vi "zad4.vi"() -> ()   [LabVIEW 2017]
panel:
  in  "Tryb awaryjny":bool
  in  "stop":bool
  out "Lampa Uliczna":cluster{"1":bool, "2":bool, "3":bool}
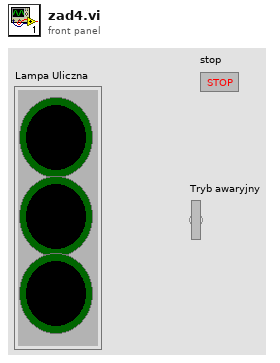
[diagram p1: front panel]
types:
  T1 = cluster{"1":bool, "2":bool, "3":bool, "2":bool, "2":bool, "2":bool, "2":bool, "2":bool}
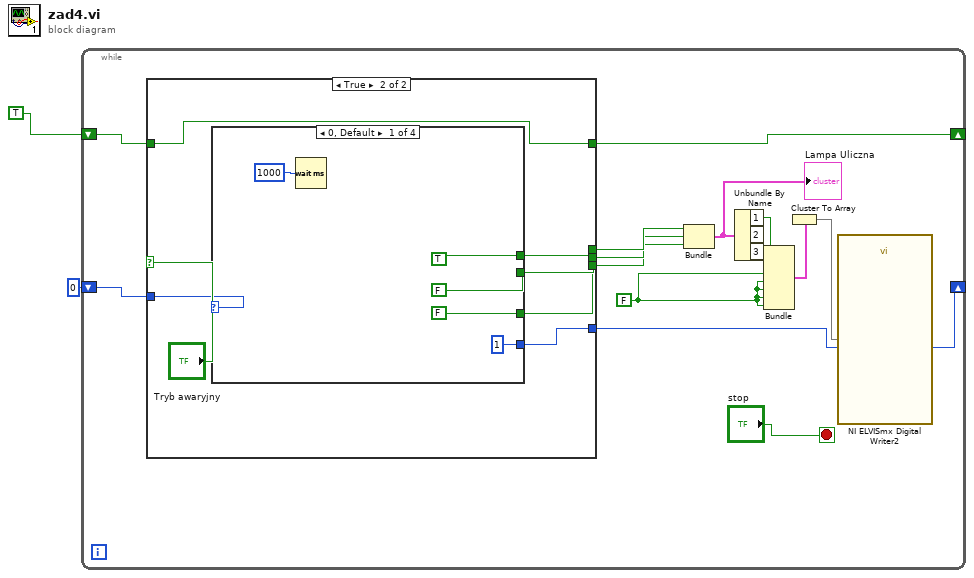
[diagram p0: block diagram]
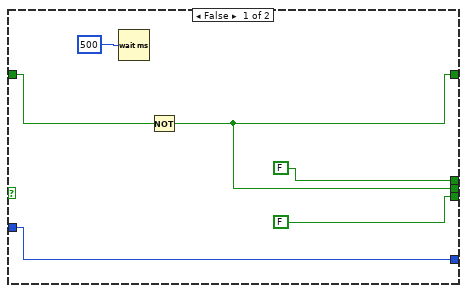
[diagram p2: hidden frame]
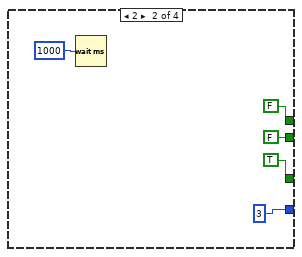
[diagram p3: hidden frame]
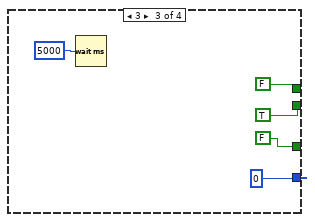
[diagram p4: hidden frame]
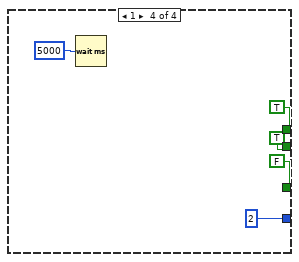
[diagram p5: hidden frame]
diagram:
  n1 = while {
    shift-right: [w10] -> _
    shift-left: 0 -> [w17]
    shift-right: [w14] -> _
    shift-left: TRUE ("2") -> [w15]
    stop <- "stop" stop-if-true
    w5 = FALSE ("2")
    n2 = case shown="True" "Tryb awaryjny" {
      tunnel: [w19 w30] -> w12
      tunnel: [FALSE ("3") w29] -> w11
      tunnel: [FALSE ("1") w28] -> w13
      tunnel: w17 -> [w22 w27]
      tunnel: [w22 w26] -> w10
      tunnel: [w19 w25] -> w14
      tunnel: w15 -> [w20 w25]
      frame False {
        n3 = Wait (ms)(milliseconds to wait=500) -> ()  [unwired: 1 out]
        n4 = Not(x=w20) -> (.not. x?=w19:bool)
      }
      frame True {
        n5 = case shown="0, Default" w27 {
          tunnel: [FALSE ("2") FALSE ("2") TRUE ("2") TRUE ("2")] -> w30
          tunnel: [FALSE ("3") TRUE ("3") FALSE ("3") FALSE ("3")] -> w29
          tunnel: [TRUE ("1") FALSE ("1") FALSE ("1") TRUE ("1")] -> w28
          tunnel: [1 3 0 2] -> w26
          frame 0, Default {
            n6 = Wait (ms)(milliseconds to wait=1000) -> ()  [unwired: 1 out]
          }
          frame 2 {
            n7 = Wait (ms)(milliseconds to wait=1000) -> ()  [unwired: 1 out]
          }
          frame 3 {
            n8 = Wait (ms)(milliseconds to wait=5000) -> ()  [unwired: 1 out]
          }
          frame 1 {
            n9 = Wait (ms)(milliseconds to wait=5000) -> ()  [unwired: 1 out]
          }
        }
      }
    }
    n10 = Bundle("1"=w13, "2"=w12, "3"=w11) -> (w9:cluster{"1":bool, "2":bool, "3":bool})  [unwired: 1 in]
    "Lampa Uliczna" <- w9
    n11 = Unbundle By Name(w9) -> ("1"=w8:bool, "2"=w7:bool, "3"=w6:bool)
    n12 = Bundle("1"=w8, "2"=w7, "3"=w6, "2"=w5, "2"=w5, "2"=w5, "2"=w5, "2"=w5) -> (w4:T1)  [unwired: 1 in]
    n13 = Cluster To Array(cluster=w4) -> (array=w3:bool[])
    n14 = call "NI ELVISmx Digital Writer2"("DO Lines"=w3) -> ()  [unwired: 18 in, 1 out]
  }
